vi "Create_empty_array.vi"(5 "Size":i32) -> (2 "Array":i32[](array[numeric]))   [LabVIEW 2019]
doc: "Create zero array of arbitray size based on size input"
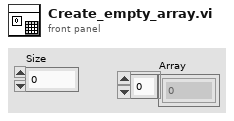
[diagram p1: front panel]
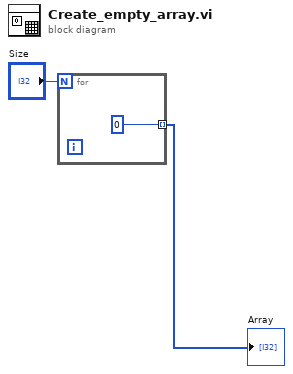
[diagram p0: block diagram]
diagram:
  n1 = for {
    N: "Size" -> [_]
    tunnel: [0] -> w2 mode=indexing
  }
  "Array" <- w2
